vi "DEV example.vi"() -> ()   [LabVIEW 2018, in "Database.lvlib"]
uses:
  Database.lvlib
  <vilib>/addons/database/Auxilliary.llb/DB Tools DataTypes.ctl
  <vilib>/addons/database/NI_Database_API.lvlib
panel:
  out "Column Information":T2(array[cluster])
  out "Column Names":string[](array[string])
  in  "Error In":errorcluster
  out "Error Out":errorcluster
  out "Query":string
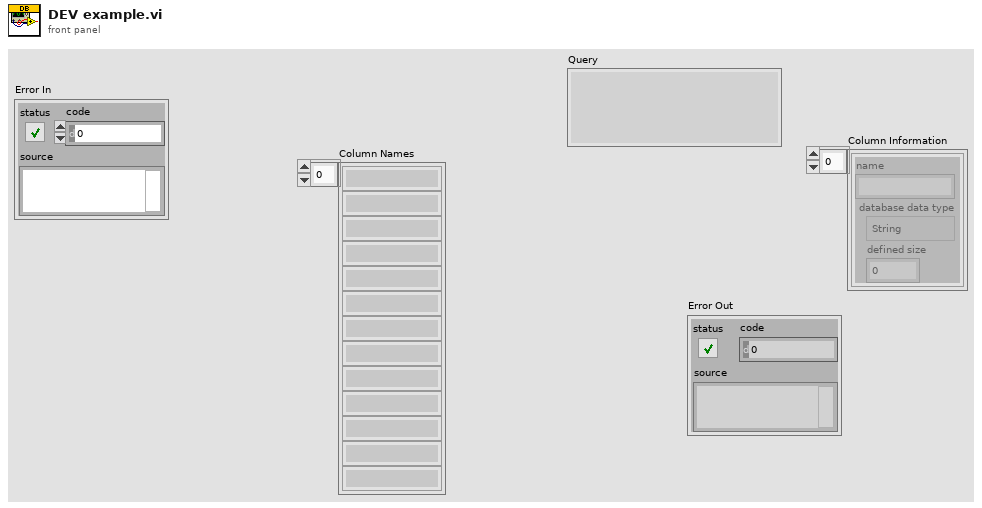
[diagram p1: front panel]
types:
  T1 = typedef "NI_Database_API.lvlib/DB Tools DataTypes.ctl" = enum16{"String", "Long (I32)", "Single (SGL)", "Double (DBL)", "Date/Time", "Binary"}
  T2 = cluster{"name":string, "database data type":T1, "defined size":i32}[]
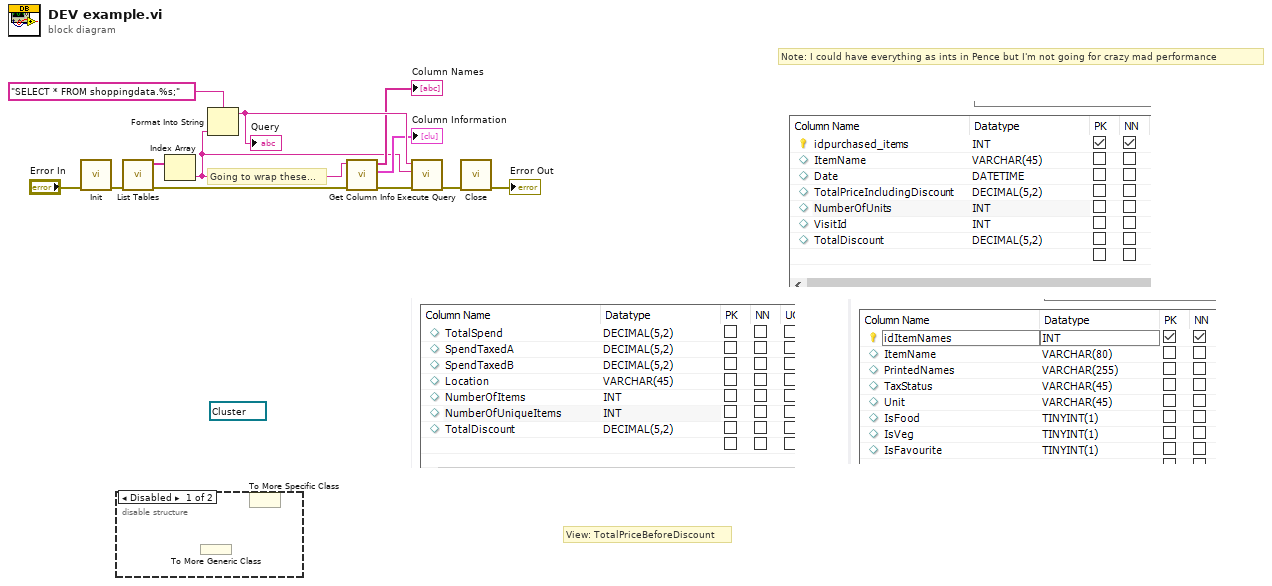
[diagram p0: block diagram]
diagram:
  (unwired) refnum<vi> refnum ("generic class reference")
  # "View: TotalPriceBeforeDiscount"
  # "Note: I could have everything as ints in Pence but I'm not going for crazy mad performance"
  # "Going to wrap these..."
  n1 = call "Init.vi"("Error In"="Error In") -> ("Error Out"=w12:errorcluster)  [unwired: 10 in]
  n2 = disable-structure shown="Disabled" {
    frame Disabled {
      n3 = To More Generic Class() -> (reference=w13:refnum<vi>)  [unwired: 1 in, 1 out]
      n4 = To More Specific Class() -> ()  [unwired: 3 in, 2 out]
    }
    frame Enabled {
    }
  }
  n5 = call "List Tables.vi"("Error In"=w12) -> ("Error Out"=w11:errorcluster, "Tables"=w10:string[])  [unwired: 9 in]
  n6 = Index Array(array=w10) -> (element=w1:string)  [unwired: 1 in]
  n7 = Format Into String(format string="SELECT * FROM shoppingdata.%s;", w1) -> (resulting string=w8:string)  [unwired: 2 in, 1 out]
  "Query" <- w8
  n8 = call "Get Column Info.vi"("Error In"=w11, "Table"=w1) -> ("Error Out"=w7:errorcluster, "Column Information"=→"Column Information":T2, "Column Names"=→"Column Names":string[])  [unwired: 7 in]
  n9 = call "Execute Query.vi"("Error In"=w7, "Table"=w1, "Query"=w8) -> ("Error Out"=w6:errorcluster)  [unwired: 6 in, 2 out]
  n10 = call "Close.vi"("Error In"=w6) -> ("Error Out"=→"Error Out":errorcluster)  [unwired: 10 in]
